vi "ReadSummaryResults_TempTest.vi"(8 "error in (no error)":errorcluster, 11 "Path":path) -> (0 "error out":errorcluster, 3 "Results":dbl[](array[numeric]))   [LabVIEW 2014]
uses:
  Excel(ActiveX)/enumOpenOrCreate.ctl
  Excel(ActiveX)/Excel(ActiveX).lvlib
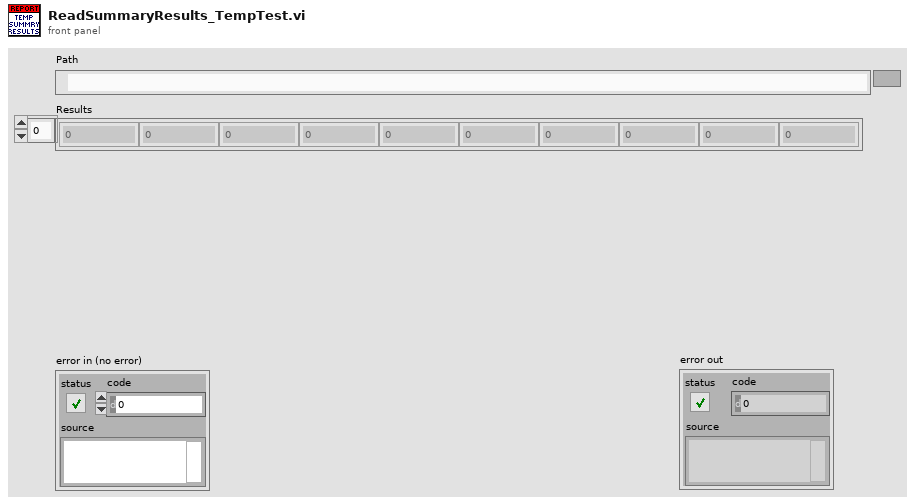
[diagram p1: front panel]
types:
  T1 = typedef "Excel(ActiveX).lvlib/enumOpenOrCreate.ctl" = enum16{"open", "open or create", "create from template"}
  T2 = typedef "Excel(ActiveX).lvlib/ExcelActiveX.ctl" = cluster{"Excel._Application":refnum<k7>, "Application open at start":bool, "Excel._Worksheet":refnum<k7>, "Workbook open at start":bool, "Excel._Workbook":refnum<k7>, "Workbook Path":path, "Worksheet Name":string, "Row":u32, "Col":u32, "Cell":string, "Workbook Name":string}
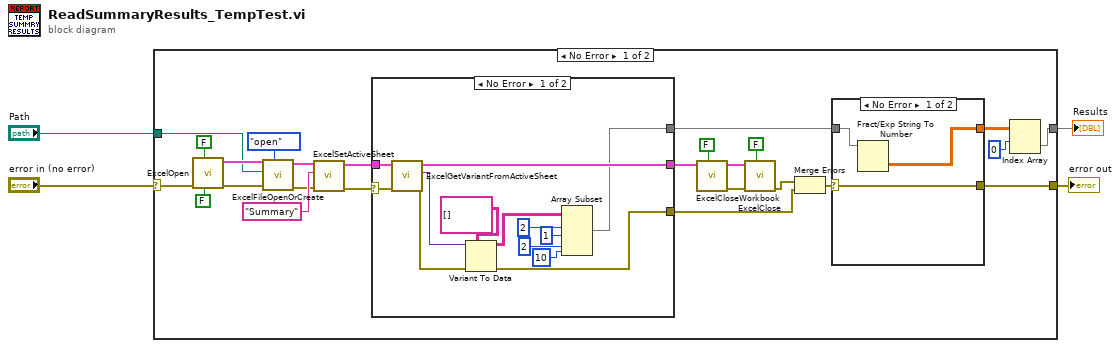
[diagram p0: block diagram]
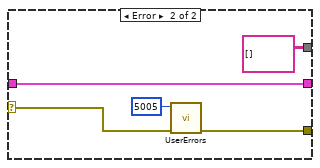
[diagram p2: hidden frame]
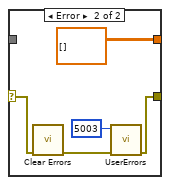
[diagram p3: hidden frame]
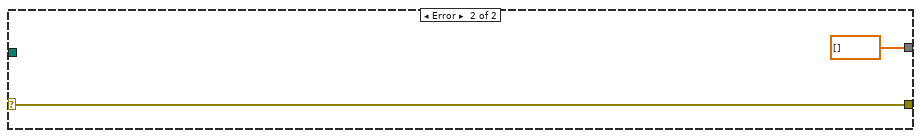
[diagram p4: hidden frame]
diagram:
  n1 = case shown="No Error" "error in (no error)" {
    selector: "error in (no error)" -> [w27 w57]
    tunnel: [w16 w57] -> w3
    tunnel: "Path" -> [w23 _]
    tunnel: [w5 dbl[] []] -> w1
    frame No Error {
      n2 = call "ExcelOpen.vi"("Run Minimized (f)"=FALSE, "Excel visible? (t)"=FALSE, "error in (no error)"=w27) -> ("error out"=w25:errorcluster, "ExcelActiveX"=w24:T2)  [unwired: 7 in]
      n3 = call "ExcelFileOpenOrCreate.vi"("Open or Create"=enumOpenOrCreate."open", "error in (no error)"=w25, "Excel file name and path"=w23, "ExcelActiveX in"=w24) -> ("error out"=w21:errorcluster, "ExcelActiveX out"=w20:T2)  [unwired: 6 in]
      n4 = call "ExcelSetActiveSheet.vi"("error in (no error)"=w21, "Sheet Name"="Summary", "ExcelActiveX in"=w20) -> ("error out"=w13:errorcluster, "ExcelActiveX  out"=w15:T2)  [unwired: 7 in]
      n5 = case shown="No Error" w13 {
        selector: w13 -> [w40 w45]
        tunnel: w15 -> [w42 w47]
        tunnel: [w41 w47] -> w10
        tunnel: [w36 w44] -> w14
        tunnel: [w30 string[][] []] -> w12
        frame No Error {
          n6 = call "ExcelGetVariantFromActiveSheet.vi"("error in (no error)"=w40, "ExcelActiveX  in"=w42) -> ("error out"=w37:errorcluster, "VariantOut"=w39:variant, "ExcelActiveX  out"=w41:T2)  [unwired: 7 in]
          n7 = Variant To Data(error in=w37, type=string[][] [], Variant=w39) -> (data=w35:string[][], error out=w36:errorcluster)
          n8 = Array Subset(array=w35, index (row)=2 ("index"), length (row)=1 ("length"), index (col)=2 ("index"), length (col)=10 ("index")) -> (w30:string[][])
        }
        frame Error {
          n9 = call "UserErrors.vi"("error in (no error)"=w45, "[error code] (0)"=5005) -> ("error out"=w44:errorcluster)  [unwired: 9 in]
        }
      }
      n10 = call "ExcelCloseWorkbook.vi"("Save"=FALSE, "ExcelActiveX"=w10) -> ("error out"=w8:errorcluster, "ExcelActiveX"=w9:T2)  [unwired: 8 in]
      n11 = call "ExcelClose.vi"("Leave Open (f)"=FALSE, "error in (no error)"=w8, "ExcelActiveX in"=w9) -> ("error out"=w19:errorcluster)  [unwired: 7 in, 1 out]
      n12 = Merge Errors(w19, w14) -> (w17:errorcluster)
      n13 = case shown="No Error" w17 {
        selector: w17 -> [w50 w55]
        tunnel: [w50 w53] -> w16
        tunnel: w12 -> [w49 _]
        tunnel: [w48 dbl[][] []] -> w11
        frame No Error {
          n14 = Fract/Exp String To Number(string=w49) -> (number=w48:dbl[][])  [unwired: 3 in, 1 out]
        }
        frame Error {
          n15 = call <vilib>:"Clear Errors.vi"("error in (no error)"=w55) -> ("error out"=w54:errorcluster)  [unwired: 5 in, 1 out]
          n16 = call "UserErrors.vi"("error in (no error)"=w54, "[error code] (0)"=5003) -> ("error out"=w53:errorcluster)  [unwired: 9 in]
        }
      }
      n17 = Index Array(array=w11, index (row)=0 ("disabled index (col)")) -> (element=w5:dbl[])  [unwired: 1 in]
    }
    frame Error {
    }
  }
  "error out" <- w3
  "Results" <- w1
